vi "Update Velocity.vi"(9 "Hit Lower Boundary?":bool, 10 "Hit Upper Boundary?":bool, 11 "Velocity":dbl) -> (3 "Updated Velocity":dbl)   [LabVIEW 2015]
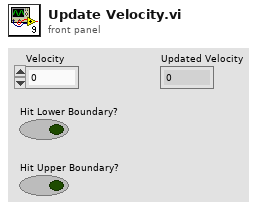
[diagram p1: front panel]
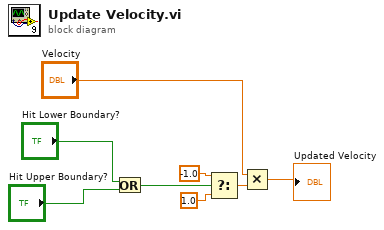
[diagram p0: block diagram]
diagram:
  n1 = Or(x="Hit Lower Boundary?", y="Hit Upper Boundary?") -> (x .or. y?=w8:bool)
  n2 = Select(t=-1.0, s=w8, f=1.0) -> (s? t:f=w1:dbl)
  n3 = Multiply(x="Velocity", y=w1) -> (x*y=→"Updated Velocity":dbl)
